vi "exportMessage.vi"(7 "path in":path=path "C:/dev/Hexagon-VTD-Custom-Device/Libraries/VC.dll", 8 "error in (no error)":errorcluster, 10 "dataOut":u8[](array[numeric]), 11 "builderHandle in":u64) -> (0 "error out":errorcluster, 2 "dataOut":u8[](array[numeric]), 3 "builderHandle out":u64)   [LabVIEW 2023, in "RDB.lvlib"]
uses:
  RDB.lvlib
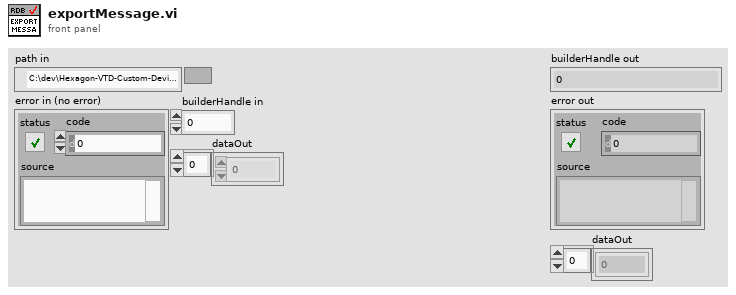
[diagram p1: front panel]
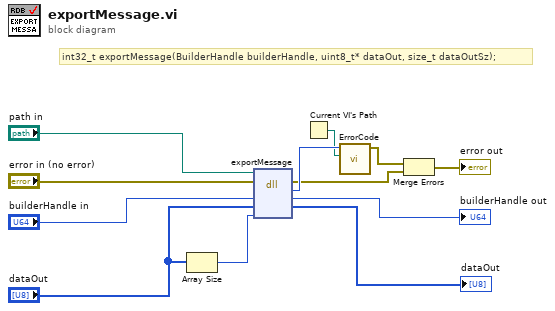
[diagram p0: block diagram]
diagram:
  # "int32_t exportMessage(BuilderHandle builderHandle, uint8_t* dataOut, size_t dataOutSz);"
  n1 = Array Size(array="dataOut") -> (size(s)=w2:i32)
  n2 = dll-call lib="C:/dev/Hexagon-VTD-Custom-Device/Libraries/libVC.dll" fn="exportMessage"(path in="path in", error in="error in (no error)", "builderHandle"="builderHandle in", "dataOut"="dataOut", "dataOutSz"=w2) -> (error out=w7:errorcluster, "return type"=w9:i32, "builderHandle"=→"builderHandle out":u64, "dataOut"=→"dataOut":u8[])  [unwired: 2 in, 1 out]
  n3 = Current VI's Path() -> (path=w4:path)
  n4 = call "ErrorCode.vi"("parent VI path"=w4, "return type"=w9) -> ("error out"=w8:errorcluster)  [unwired: 9 in]
  n5 = Merge Errors(w8, w7) -> (→"error out":errorcluster)
